vi "Hide Unused.vi"(5 "Connector Type":T1, 7 "Hide unused":bool, 12 "Connector array":refnum<vi>[](array[refnum])) -> ()   [LabVIEW 2020, in "PXISlot.xctl"]
uses:
  PXISlot.xctl
  Connector Type.ctl
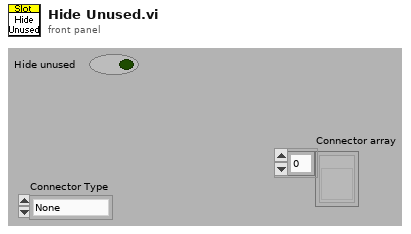
[diagram p1: front panel]
types:
  T1 = typedef "Connector Type.ctl" = enum16{"None", "PXI-4461", "BNC-2110", "BNC-2090", "PXIe-4463", "PXIe-4464"}
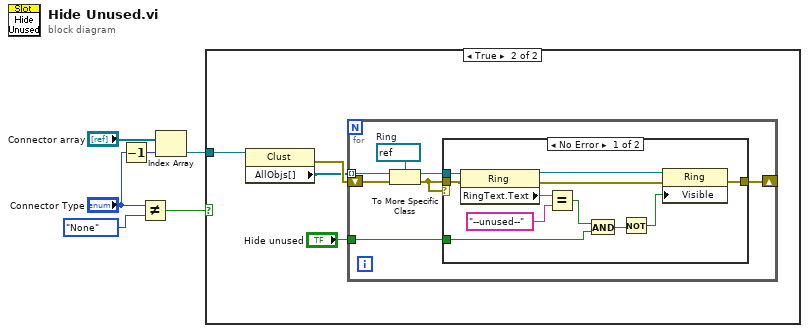
[diagram p0: block diagram]
diagram:
  n1 = Decrement(x="Connector Type") -> (x-1=w2:T1)
  n2 = Not Equal?(x="Connector Type", y=Connector_Type."None") -> (x != y?=w5:bool)
  n3 = Index Array(array="Connector array", index=w2) -> (element=w3:refnum<vi>)
  n4 = case shown="True" w5 {
    tunnel: w3 -> [_ w7]
    frame False {
    }
    frame True {
      n5 = property class="Clust"(reference=w7) -> (error out=w9:errorcluster, "AllObjs[]"=w8:refnum<vi>[])  [unwired: 1 in, 1 out]
      n6 = for {
        tunnel: w8 -> [w12] mode=indexing
        tunnel: "Hide unused" -> [w16]
        shift-right: [w15] -> _
        shift-left: w9 -> [w13]
        w17 = refnum<vi> refnum  # Ring
        n7 = To More Specific Class(target class=w17, reference=w12, error in=w13) -> (specific class reference=w11:refnum<vi>, error out=w14:errorcluster)
        n8 = case shown="No Error" w14 {
          tunnel: w11 -> [w28 _]
          tunnel: w16 -> [w24 _]
          tunnel: w14 -> [w22 _]
          tunnel: [w20 _] -> w15
          frame No Error {
            n9 = property class="Ring"(reference=w28, error in=w22) -> (reference out=w25:refnum<vi>, error out=w21:errorcluster, "RingText.Text"=w27:string)
            n10 = Equal?(x=w27, y="--unused--") -> (x = y?=w19:bool)
            n11 = And(x=w19, y=w24) -> (x .and. y?=w23:bool)
            n12 = Not(x=w23) -> (.not. x?=w18:bool)
            n13 = property class="Ring"(reference=w25, error in=w21, "Visible"=w18) -> (error out=w20:errorcluster)  [unwired: 1 out]
          }
          frame Error {
          }
        }
      }
    }
  }
